vi "Porcent Acquired.vi"(8 "error in (no error)":errorcluster, 11 "CCDCamera in":refnum<class "CCDCamera.lvclass">) -> (0 "error out":errorcluster, 2 "% Acquired":dbl, 3 "CCDCamera out":refnum<class "CCDCamera.lvclass">)   [LabVIEW 2018, in "CCDCamera.lvclass"]
doc: "This VI returns the percentage of the acquisitiong (FLOAT) of the current image."
uses:
  CCDCamera.lvclass
  CCDCamera.lvclass/CCDCamera.ctl
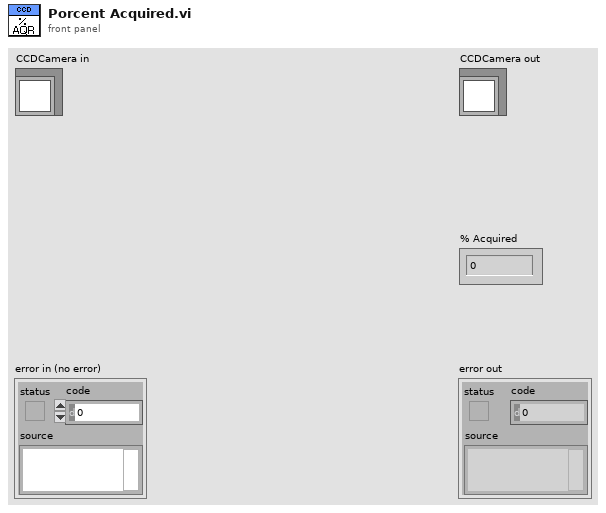
[diagram p1: front panel]
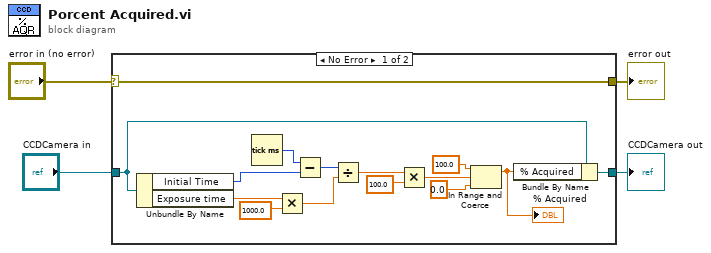
[diagram p0: block diagram]
diagram:
  n1 = case shown="No Error" "error in (no error)" {
    selector: "error in (no error)" -> [w19 w21]
    tunnel: [w19 w21] -> w3
    tunnel: [w8 w20] -> w1
    tunnel: "CCDCamera in" -> [w9 w20]
    frame No Error {
      n2 = Unbundle By Name(w9) -> ("Initial Time"=w7:u32, "Exposure time"=w18:dbl)
      n3 = Tick Count (ms)() -> (millisecond timer value=w6:u32)
      n4 = Multiply(x=w18, y=1000.0) -> (x*y=w16:dbl)
      n5 = Subtract(x=w6, y=w7) -> (x-y=w15:u32)
      n6 = Divide(x=w15, y=w16) -> (x/y=w14:dbl)
      n7 = Multiply(x=w14, y=100.0) -> (x*y=w10:dbl)
      n8 = In Range and Coerce(upper limit=100.0 ("y"), x=w10, lower limit=0.0) -> (coerced(x)=w5:dbl)  [unwired: 1 out]
      "% Acquired" <- w5
      n9 = Bundle By Name(cluster=w9, "% Acquired"=w5) -> (w8:refnum<class "CCDCamera.lvclass">)
    }
    frame Error {
    }
  }
  "error out" <- w3
  "CCDCamera out" <- w1
